vi "TwoBallAutoRTv2.vi"   [LabVIEW 2015]
uses:
  <vilib>/Rock Robotics/WPI/DriverStation/WPI_DriverStationRobotMode2.ctl
  Utilities/MotorPositionGlobals.vi
  Utilities/AutoVars.vi
  TwoBallAutoGlobals.vi
  navx-mxp/labview/navX Library v2/navX Library v2.lvlib
types:
  T1 = enum16{"WaitForInput", "StartIntake", "LowerArm", "IntakeBall", "TurnAndZeroEnc", "DriveForward", "RecordGyro", "TargetAndLoad", "Shoot", "TurnBack", "BackUpAndIntake", "IntakeBall2", "DriveForward2", "TargetAndLoad2", "Shoot2", "End"}
  T2 = typedef "WPI_DriverStationRobotMode2.ctl" = enum16{"Autonomous Disabled", "Autonomous Enabled", "Teleop Disabled", "Teleop Enabled", "Disconnected", "Finish", "Test Disabled", "Test Enabled", "Emergency Stopped"}
  T3 = typedef "navX Library v2.lvlib/Z900_navX_DeviceTypeDef.ctl" = cluster{"Interface":cluster{"Protocol":T4, "Update Rate (4Hz-100Hz)":u8, "navX Open TypeDef":variant}, "Notify Packet":refnum<notifier>, "Loop VI Refnum":refnum<vi>, "Ready to Close Occurrence Refnum":refnum<k4>}
  T4 = typedef "navX Library v2.lvlib/Z900_navX_ProtocolTypeDef.ctl" = enum16{"SERIAL", "I2C", "SPI"}
  T5 = cluster{"Yaw":dbl, "Roll":dbl, "Pitch":dbl, "Heading":dbl, "Fused Heading":dbl}
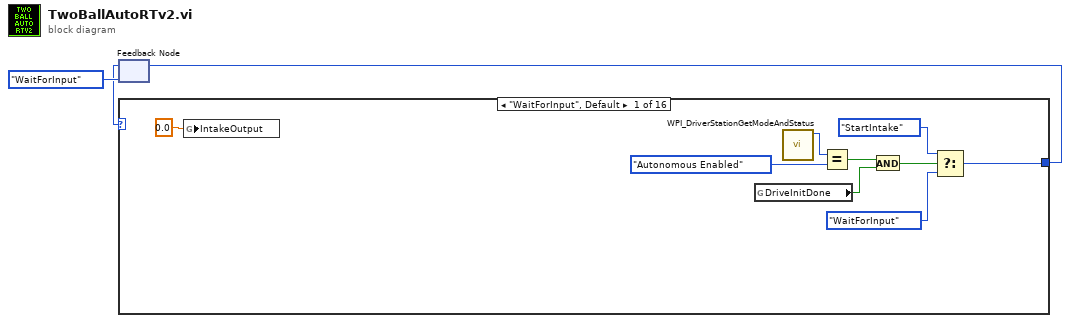
[diagram p0: block diagram]
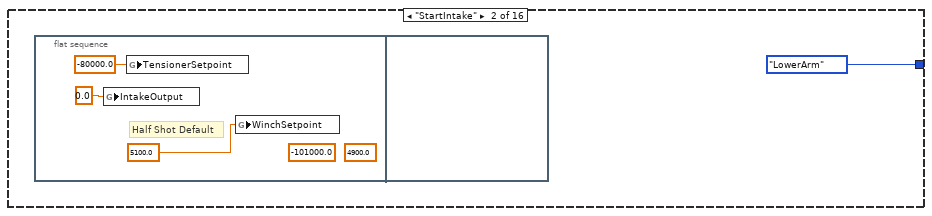
[diagram p2: hidden frame]
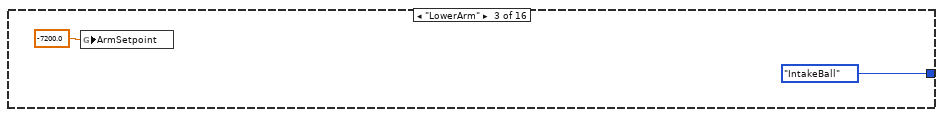
[diagram p3: hidden frame]
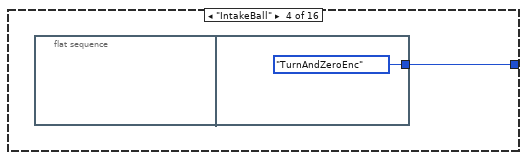
[diagram p4: hidden frame]
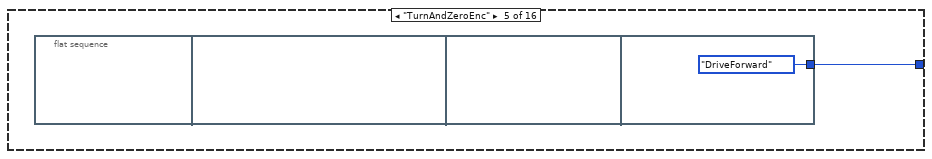
[diagram p5: hidden frame]
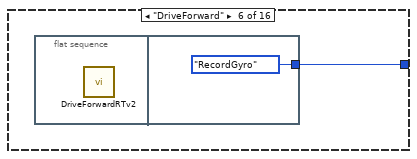
[diagram p6: hidden frame]
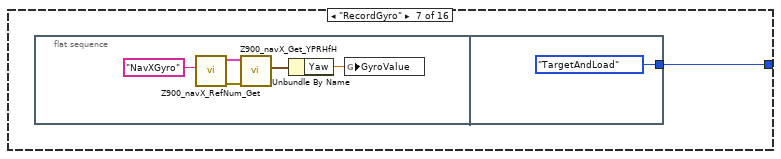
[diagram p7: hidden frame]
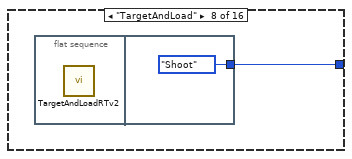
[diagram p8: hidden frame]
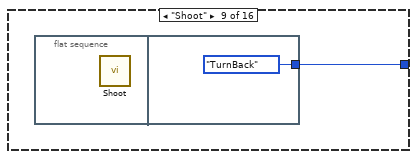
[diagram p9: hidden frame]
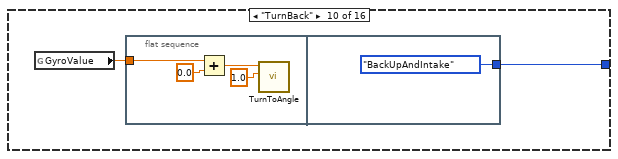
[diagram p10: hidden frame]
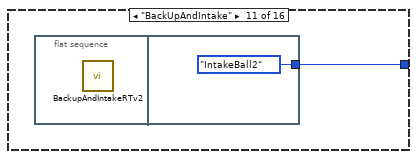
[diagram p11: hidden frame]
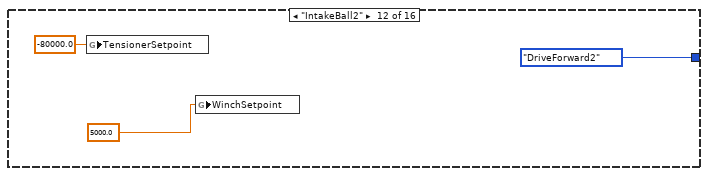
[diagram p12: hidden frame]
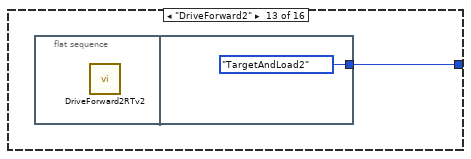
[diagram p13: hidden frame]
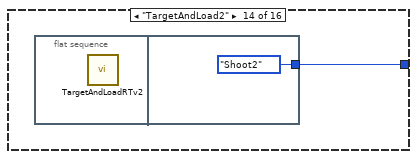
[diagram p14: hidden frame]
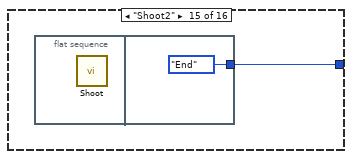
[diagram p15: hidden frame]
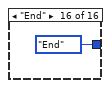
[diagram p16: hidden frame]
diagram:
  n1 = feedback #1(T1."WaitForInput" ("Enum")) -> (w1:T1)
  n2 = case shown="\"WaitForInput\", Default" w1 {
    tunnel: [w5 T1."LowerArm" ("Enum") T1."IntakeBall" ("Enum") w19 w21 w23 w25 w32 w34 w36 w43 T1."DriveForward2" ("Enum") w48 w50 w52 T1."End" ("Enum")] -> w3
    frame "WaitForInput", Default {
      n3 = global write "MotorPositionGlobals.vi" "IntakeOutput"(0.0 ("IntakeOutput")) -> ()
      n4 = global read "AutoVars.vi" "DriveInitDone"() -> (w9:bool)
      n5 = call <vilib>:"WPI_DriverStationGetModeAndStatus.vi"() -> ("Robot Mode"=w12:T2)  [unwired: 10 in, 1 out]
      n6 = Equal?(x=w12, y=WPI_DriverStationRobotMode2."Autonomous Enabled" ("Robot Mode")) -> (x = y?=w10:bool)
      n7 = And(x=w10, y=w9) -> (x .and. y?=w8:bool)
      n8 = Select(t=T1."StartIntake" ("Enum"), s=w8, f=T1."WaitForInput" ("Enum")) -> (s? t:f=w5:T1)
    }
    frame "StartIntake" {
      n9 = flat-sequence {
        frame #0 {
          (unwired) 4900.0 ("WinchPosition")
          (unwired) -101000.0 ("TensionerSetpoint")
          # "Half Shot Default"
          n10 = global write "MotorPositionGlobals.vi" "IntakeOutput"(0.0 ("IntakeOutput")) -> ()
          n11 = global write "MotorPositionGlobals.vi" "TensionerSetpoint"(-80000.0 ("TensionerSetpoint")) -> ()
          n12 = global write "MotorPositionGlobals.vi" "WinchSetpoint"(5100.0 ("WinchPosition")) -> ()
        }
        frame #1 {
        }
      }
    }
    frame "LowerArm" {
      n13 = global write "MotorPositionGlobals.vi" "ArmSetpoint"(-7200.0 ("ArmSetpoint")) -> ()
    }
    frame "IntakeBall" {
      n14 = flat-sequence {
        tunnel: [T1."TurnAndZeroEnc" ("Enum")] -> w19
        frame #0 {
        }
        frame #1 {
        }
      }
    }
    frame "TurnAndZeroEnc" {
      n15 = flat-sequence {
        tunnel: [T1."DriveForward" ("Enum")] -> w21
        frame #0 {
        }
        frame #1 {
        }
        frame #2 {
        }
        frame #3 {
        }
      }
    }
    frame "DriveForward" {
      n16 = flat-sequence {
        tunnel: [T1."RecordGyro" ("Enum")] -> w23
        frame #0 {
          n17 = call "DriveForwardRTv2.vi"() -> ()  [unwired: 12 in]
        }
        frame #1 {
        }
      }
    }
    frame "RecordGyro" {
      n18 = flat-sequence {
        tunnel: [T1."TargetAndLoad" ("Enum")] -> w25
        frame #0 {
          n19 = call "Z900_navX_RefNum_Get.vi"("refnum name"="NavXGyro") -> ("error out"=w29:errorcluster, "navX Device"=w30:T3)  [unwired: 9 in]
          n20 = call "Z900_navX_Get_YPRHfH.vi"("error in (no error)"=w29, "navX Device"=w30) -> ("YRPHfH"=w27:T5)  [unwired: 6 in, 3 out]
          n21 = Unbundle By Name(w27) -> ("Yaw"=w26:dbl)
          n22 = global write "TwoBallAutoGlobals.vi" "GyroValue"(w26) -> ()
        }
        frame #1 {
        }
      }
    }
    frame "TargetAndLoad" {
      n23 = flat-sequence {
        tunnel: [T1."Shoot" ("Enum")] -> w32
        frame #0 {
          n24 = call "TargetAndLoadRTv2.vi"() -> ()  [unwired: 1 in]
        }
        frame #1 {
        }
      }
    }
    frame "Shoot" {
      n25 = flat-sequence {
        tunnel: [T1."TurnBack" ("Enum")] -> w34
        frame #0 {
          n26 = call "Shoot.vi"() -> ()  [unwired: 12 in]
        }
        frame #1 {
        }
      }
    }
    frame "TurnBack" {
      n27 = global read "TwoBallAutoGlobals.vi" "GyroValue"() -> (w37:dbl)
      n28 = flat-sequence {
        tunnel: w37 -> [w40]
        tunnel: [T1."BackUpAndIntake" ("Enum")] -> w36
        frame #0 {
          n29 = Add(x=w40, y=0.0) -> (x+y=w39:dbl)
          n30 = call "TurnToAngle.vi"("AllowedDeviation"=1.0, "GyroValue"=w39) -> ()  [unwired: 10 in]
        }
        frame #1 {
        }
      }
    }
    frame "BackUpAndIntake" {
      n31 = flat-sequence {
        tunnel: [T1."IntakeBall2" ("Enum")] -> w43
        frame #0 {
          n32 = call "BackupAndIntakeRTv2.vi"() -> ()  [unwired: 2 in]
        }
        frame #1 {
        }
      }
    }
    frame "IntakeBall2" {
      n33 = global write "MotorPositionGlobals.vi" "TensionerSetpoint"(-80000.0 ("TensionerSetpoint")) -> ()
      n34 = global write "MotorPositionGlobals.vi" "WinchSetpoint"(5000.0 ("WinchPosition")) -> ()
    }
    frame "DriveForward2" {
      n35 = flat-sequence {
        tunnel: [T1."TargetAndLoad2" ("Enum")] -> w48
        frame #0 {
          n36 = call "DriveForward2RTv2.vi"() -> ()  [unwired: 2 in]
        }
        frame #1 {
        }
      }
    }
    frame "TargetAndLoad2" {
      n37 = flat-sequence {
        tunnel: [T1."Shoot2" ("Enum")] -> w50
        frame #0 {
          n38 = call "TargetAndLoadRTv2.vi"() -> ()  [unwired: 1 in]
        }
        frame #1 {
        }
      }
    }
    frame "Shoot2" {
      n39 = flat-sequence {
        tunnel: [T1."End" ("Enum")] -> w52
        frame #0 {
          n40 = call "Shoot.vi"() -> ()  [unwired: 12 in]
        }
        frame #1 {
        }
      }
    }
    frame "End" {
    }
  }
  n41 = feedback-in #1(w3) -> ()
